vi "Read Config.vi"(8 "error in (no error)":errorcluster) -> (0 "error out":errorcluster, 3 "SignalConfig":T1={"VPP"=0, "Frecuency"=50.0, "Offset"=0.0, "signal type"=enum."Sine Wave"})   [LabVIEW 2020, in "DataBase.lvlib"]
uses:
  DataBase.lvlib
  Acquisition/SignalConfig--cluster.ctl
  <vilib>/drjdpowell/SQLite Library/SQL Connection/Open (path).vi
  <vilib>/drjdpowell/SQLite Library/SQL Connection/Open (string).vi
  <vilib>/AdvancedString/Path To Command Line String.vi
  <vilib>/drjdpowell/SQLite Library/SQL Connection/Execute SQL (1D String).vi
  <vilib>/drjdpowell/SQLite Library/SQL Connection/Connection.lvclass
  <vilib>/drjdpowell/SQLite Library/SQLite.lvlib
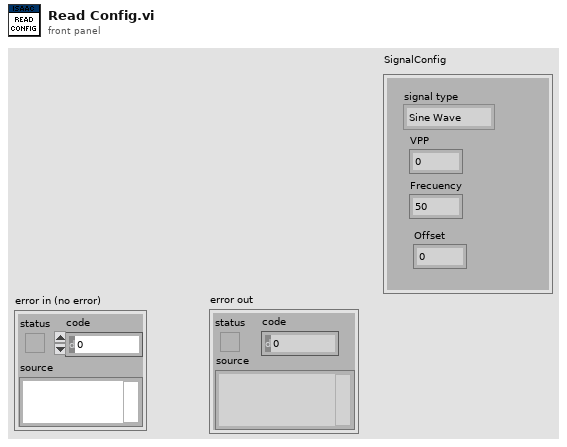
[diagram p1: front panel]
types:
  T1 = typedef "SignalConfig--cluster.ctl" = cluster{"VPP":i32, "Frecuency":dbl, "Offset":dbl, "signal type":enum16{"Sine Wave", "Triangle Wave", "Square Wave", "Sawtooth Wave"}}
  T2 = enum16{"Sine Wave", "Triangle Wave", "Square Wave", "Sawtooth Wave"}
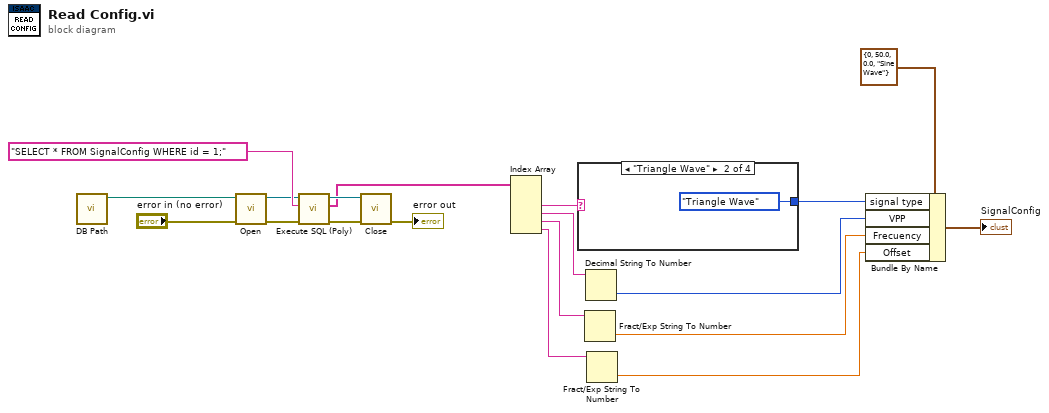
[diagram p0: block diagram]
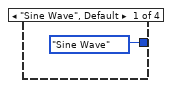
[diagram p2: hidden frame]
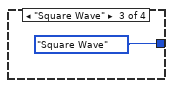
[diagram p3: hidden frame]
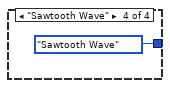
[diagram p4: hidden frame]
diagram:
  n1 = call "DB Path.vi"() -> ("appended path"=w15:path)  [unwired: 11 in]
  n2 = call-poly <vilib>:"Open.vi"("error in (no error)"="error in (no error)", "db file"=w15) -> ("error out"=w19:errorcluster, "SQLite Connection"=w13:refnum<class "Connection.lvclass">)  [unwired: 8 in]
  n3 = call-poly <vilib>:"Execute SQL (Poly).vi"("error in (no error)"=w19, "SQL"="SELECT * FROM SignalConfig WHERE id = 1;", "SQLite Connection in"=w13) -> ("error out"=w18:errorcluster, "Result Set"=w11:string[], "SQLite Connection"=w12:refnum<class "Connection.lvclass">)  [unwired: 5 in, 1 out]
  n4 = call-dynamic "Close.vi"("error in (no error)"=w18, "SQLite Connection in"=w12) -> ("error out"=→"error out":errorcluster)  [unwired: 9 in]
  n5 = Index Array(array=w11) -> (element #2=w10:string, element #3=w7:string, element #4=w9:string, element #5=w8:string)  [unwired: 5 in, 1 out]
  n6 = case shown="\"Triangle Wave\"" w10 {
    tunnel: [T2."Sine Wave" ("signal type") T2."Triangle Wave" ("signal type") T2."Square Wave" ("signal type") T2."Sawtooth Wave" ("signal type")] -> w4
    frame "Sine Wave", Default {
    }
    frame "Triangle Wave" {
    }
    frame "Square Wave" {
    }
    frame "Sawtooth Wave" {
    }
  }
  n7 = Fract/Exp String To Number(string=w9) -> (number=w2:dbl)  [unwired: 3 in, 1 out]
  n8 = Decimal String To Number(string=w7) -> (number=w3:i32)  [unwired: 2 in, 1 out]
  n9 = Fract/Exp String To Number(string=w8) -> (number=w1:dbl)  [unwired: 3 in, 1 out]
  n10 = Bundle By Name(cluster=T1 {"VPP"=0, "Frecuency"=50.0, "Offset"=0.0, "signal type"=enum."Sine Wave"} ("SignalConfig"), "signal type"=w4, "VPP"=w3, "Frecuency"=w2, "Offset"=w1) -> (→"SignalConfig":T1)
